vi "ADO Item Value.vi"(8 "error in (no error)":errorcluster, 11 "Item In":refnum<k7>) -> (0 "error out":errorcluster, 2 "Value":string, 3 "Item Out":refnum<k7>)   [LabVIEW 2013]
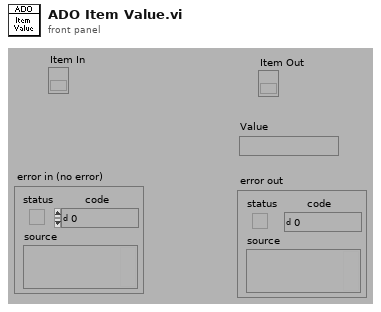
[diagram p1: front panel]
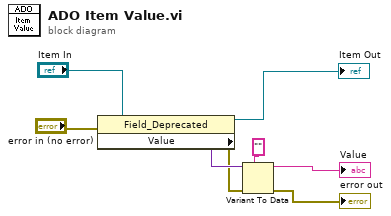
[diagram p0: block diagram]
diagram:
  n1 = property class="Field_Deprecated"(reference="Item In", error in="error in (no error)") -> (reference out=→"Item Out":refnum<k7>, error out=w3:errorcluster, "Value"=w5:variant)
  n2 = Variant To Data(error in=w3, type="", Variant=w5) -> (data=→"Value":string, error out=→"error out":errorcluster)
